vi "Markers Update.vi"(8 "error in (no error)":errorcluster, 10 "Accel Markers":string[][](array[string]), 11 "Logging in":refnum<class "Logging.lvclass">) -> (0 "error out":errorcluster, 3 "Logging out":refnum<class "Logging.lvclass">)   [LabVIEW 2020, in "Logging.lvlib" / "Logging.lvclass"]
uses:
  Logging.lvclass
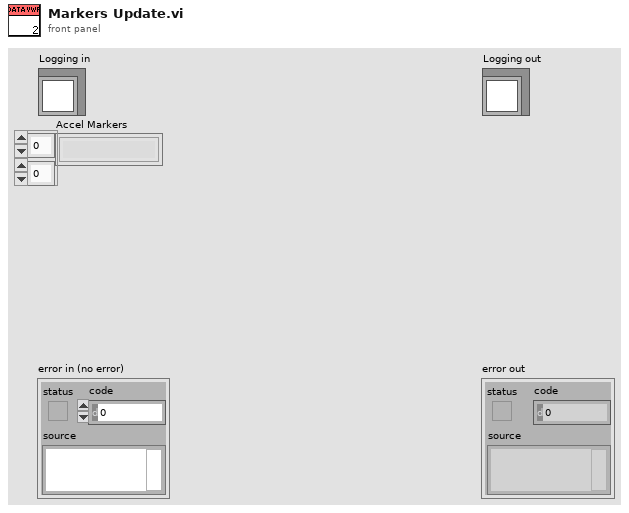
[diagram p1: front panel]
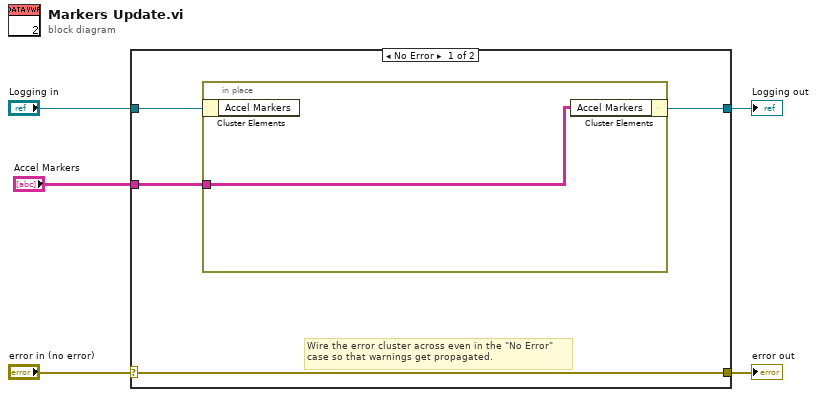
[diagram p0: block diagram]
diagram:
  n1 = case shown="No Error" "error in (no error)" {
    selector: "error in (no error)" -> [w9 w12]
    tunnel: [w9 w12] -> w4
    tunnel: [w6 w11] -> w2
    tunnel: "Logging in" -> [w8 w11]
    tunnel: "Accel Markers" -> [w7 _]
    frame No Error {
      # "Wire the error cluster across even in the \"No Error\"\ncase so that warnings get propagated."
      n2 = in-place {
        in-place-border: w7 -> [w10]
        n3 = in-place-cluster #1(w8) -> ()  [unwired: 1 out]
        n4 = in-place-cluster #1("Accel Markers"=w10) -> (w6:refnum<class "Logging.lvclass">)
      }
    }
    frame Error {
    }
  }
  "error out" <- w4
  "Logging out" <- w2
